vi "Set Channels.vi"(8 "error in (no error)":errorcluster, 9 "Trigger Source":tag, 10 "Analog Output":tag, 11 "NI Galvo in":refnum<class "A7M20.lvclass">) -> (0 "error out":errorcluster, 3 "NI Galvo out":refnum<class "A7M20.lvclass">)   [LabVIEW 2015, in "A7M20.lvclass"]
uses:
  A7M20.lvclass
  A7M20.lvclass/A7M20.ctl
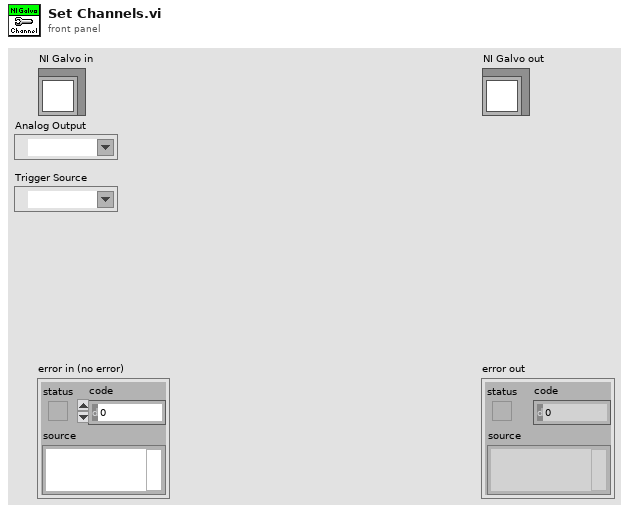
[diagram p1: front panel]
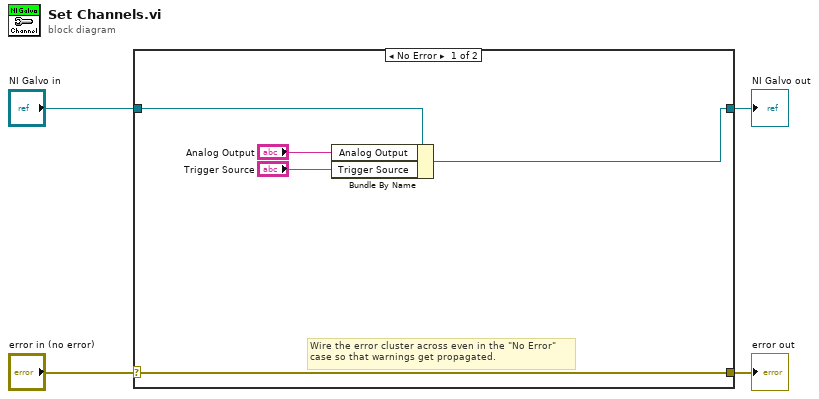
[diagram p0: block diagram]
diagram:
  n1 = case shown="No Error" "error in (no error)" {
    selector: "error in (no error)" -> [w9 w11]
    tunnel: [w9 w11] -> w3
    tunnel: [w7 w10] -> w1
    tunnel: "NI Galvo in" -> [w8 w10]
    frame No Error {
      # "Wire the error cluster across even in the \"No Error\"\ncase so that warnings get propagated."
      n2 = Bundle By Name(cluster=w8, "Analog Output"="Analog Output", "Trigger Source"="Trigger Source") -> (w7:refnum<class "A7M20.lvclass">)
    }
    frame Error {
    }
  }
  "error out" <- w3
  "NI Galvo out" <- w1
